vi "cDAQ_VI_Leo_ControlLoop.vi"() -> ()   [LabVIEW 2022 SP3]
uses:
  <vilib>/Analysis/baseanly.llb/Mean (DBL).vi
  STOP_GLOBAL.vi
  <vilib>/DAQmx/miscellaneous.llb/DAQmx Fill In Error Info.vi
  <vilib>/DAQmx/configure/timing.llb/DAQmx Timing (Sample Clock).vi
  <vilib>/DAQmx/read.llb/DAQmx Read (Analog 1D Wfm NChan NSamp).vi
  <vilib>/Analysis/NI_AALBase.lvlib
  <vilib>/addons/control/pid/NI_PID_pid.lvlib
  <vilib>/ptbypt/NI_PtbyPt.lvlib
  <vilib>/addons/control/pid/pid.llb/PID (DBL).vi
panel:
  out "Gauge":cluster{dbl, dbl}(knob) scale=0.0..10.0
  in  "Setpoint":dbl(slide) scale=0.0..10.0
  in  "Output Range":cluster{"output high":dbl, "output low":dbl}={"output high"=100.0, "output low"=-100.0} {"output low" format="%.2f"; "output high" format="%.2f"}
  in  "PID gains":T1={"proportional gain (Kc)"=1.0, "integral time (Ti, min)"=0.01, "derivative time (Td, min)"=0.0} {"derivative time (Td, min)" format="%.3f"; "integral time (Ti, min)" format="%.3f"; "proportional gain (Kc)" format="%.3f"}
  out "element 2":dbl
  out "Array 2":dbl[](array[numeric])
  out "size(s)":i32
  out "Array":dbl[](array[numeric])
  in  "rate":dbl=1000.0 format="%0.2f"
  in  "number of samples":i32=100
  in  "File Format":string
  in  "File Name Out":string
  in  "Data Collection Folder":path
  out "Temperature":dbl[](graph)
  out "Temperature":dynamicdata(graph)
  out "Thrust":dbl[](graph)
  out "Numeric 2":i32
  out "Thrust lb":dynamicdata(graph)
  in  "Types of Testing":enum32{"Test Firing", "Cold Flow Rig"}(tab)
  out "Saving Data":bool
  out "Filename Out":path
  in  "Collect Data?":bool=TRUE caption="Enable"
  in  "Collect Data? 2":bool=TRUE caption="Enable"
  out "Saving Data":bool
  out "Filename Out":path
  out "Supply Pressure PSI":dynamicdata(graph)
  out "4th Channel NI 9219":dynamicdata(graph)
  out "Mass Flow":dbl[](graph)
  out "Mass Flow L/min":dynamicdata(graph)
  out "Chamber Pressure":dbl[](graph)
  out "Supply Pressure":dbl[](graph)
  out "Chamber Pressure PSI":dynamicdata(graph)
  # "DATA LOGGING INFORMATION"
  # "ANALOG VOLTAGE OUTPUT"
  # "RESULTS"
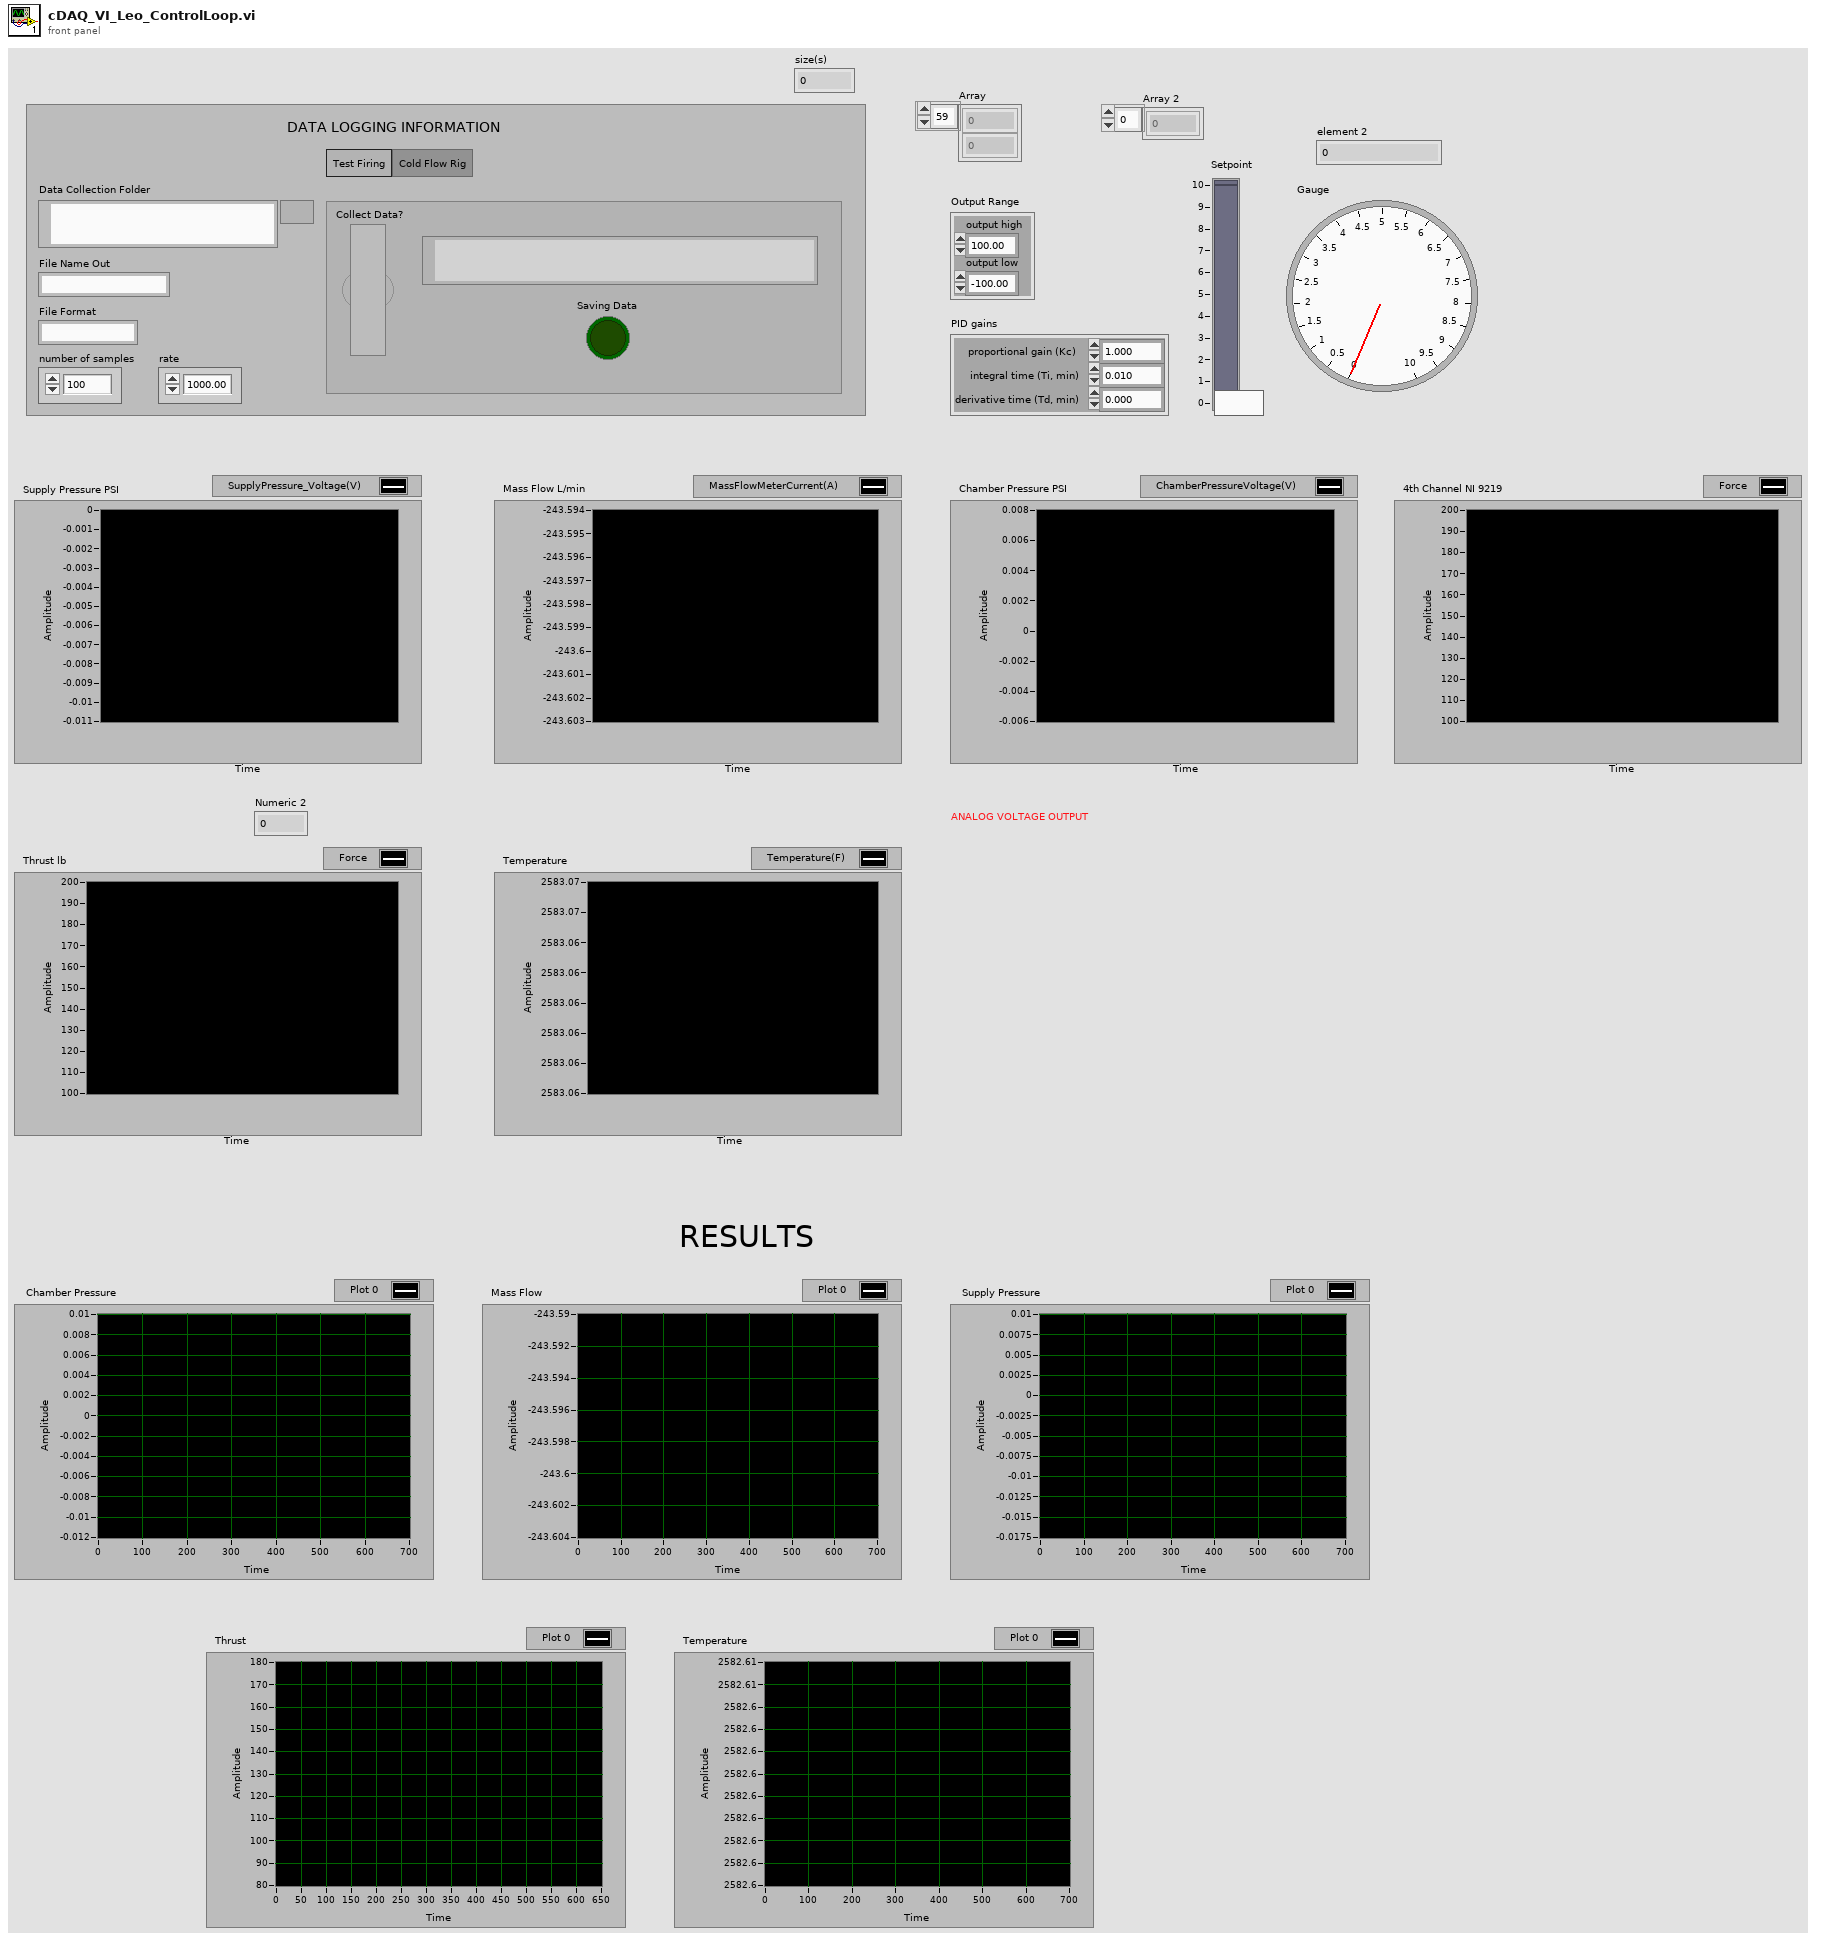
[diagram p1: front panel]
types:
  T1 = cluster{"proportional gain (Kc)":dbl, "integral time (Ti, min)":dbl, "derivative time (Td, min)":dbl}
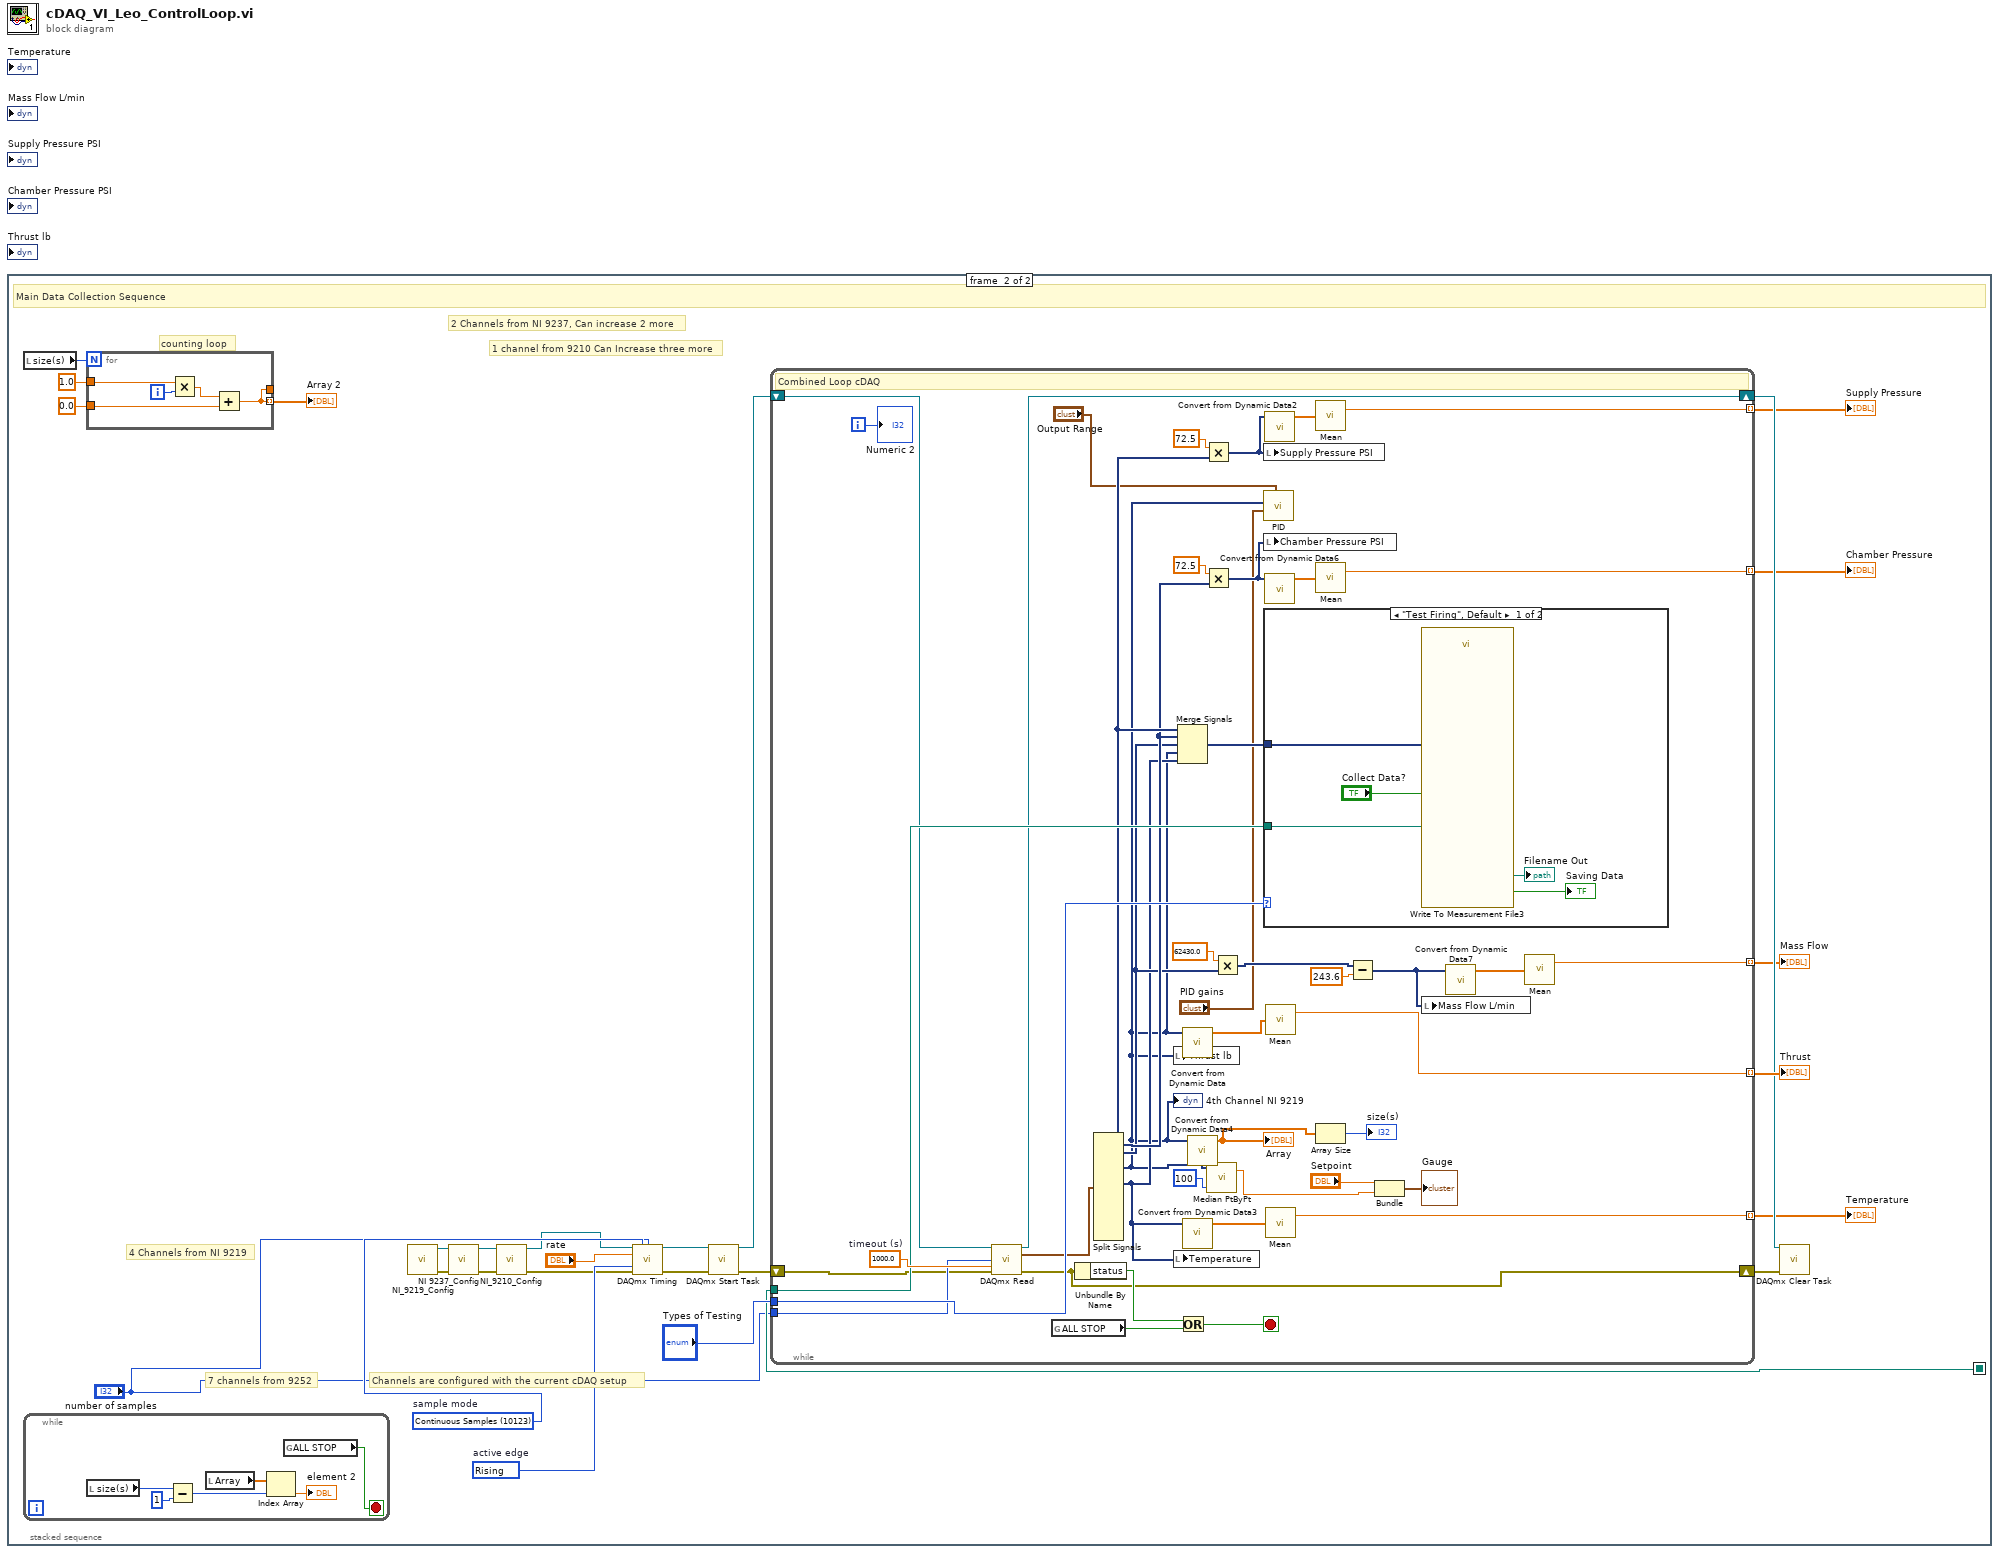
[diagram p0: block diagram]
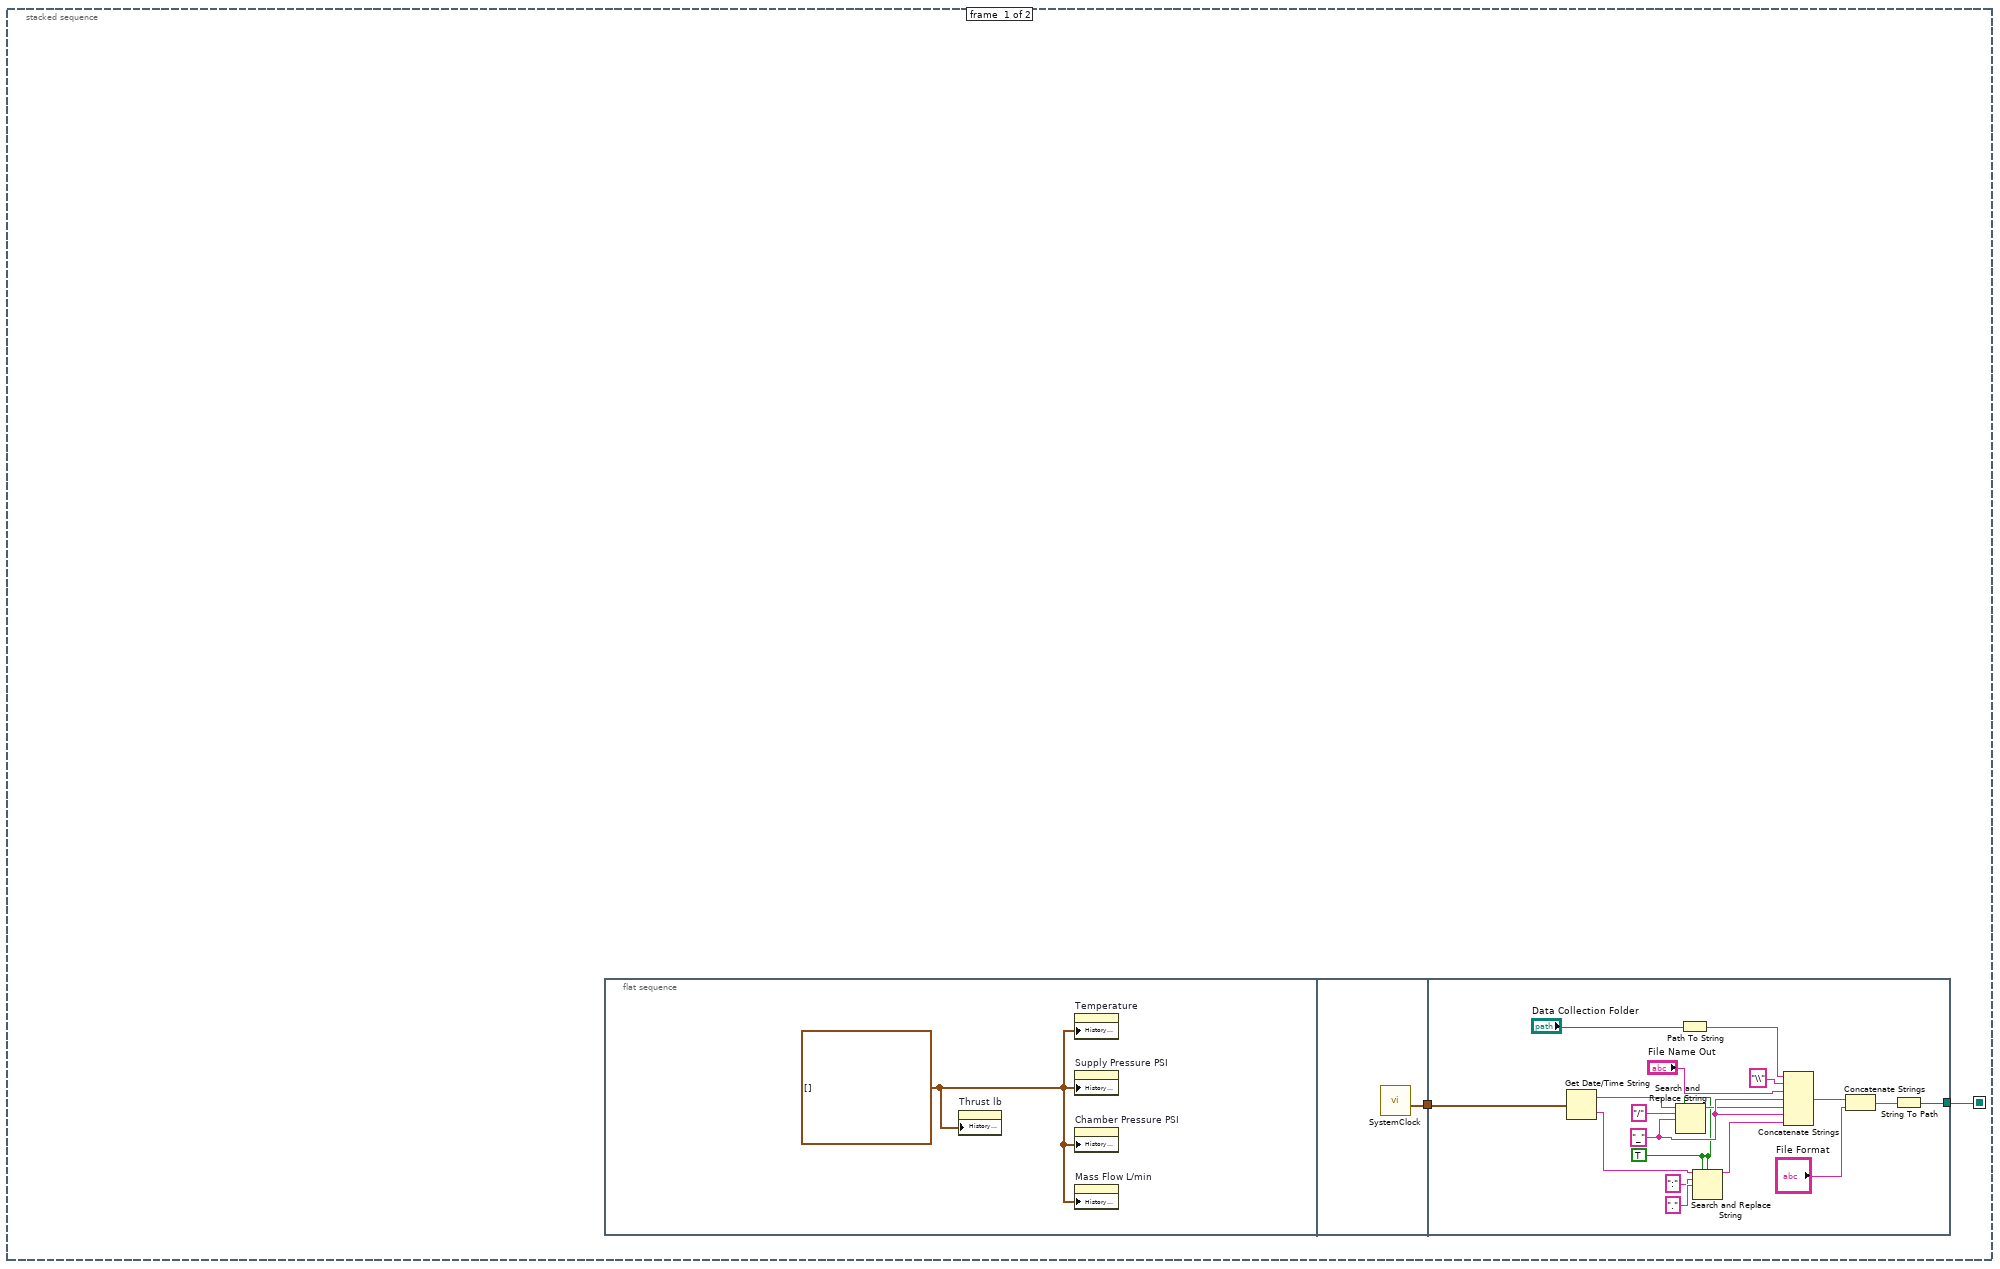
[diagram p2: hidden frame]
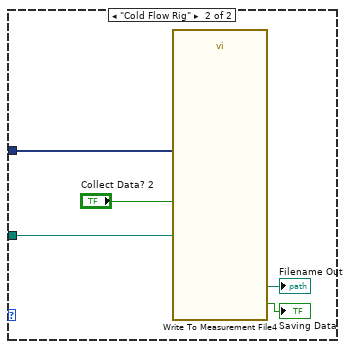
[diagram p3: hidden frame]
diagram:
  n1 = stacked-sequence {
    seq-local: [w1 _] -> [_ w47]
    frame #0 {
      n2 = flat-sequence {
        tunnel: [w4] -> w2
        tunnel: w2 -> [w11]
        tunnel: [w10] -> w1
        frame #0 {
          w3 = waveform(dbl)[] []
          n3 = property on="Thrust lb" class="WFChart (strict)"("History Data"=w3) -> ()  [unwired: 2 in, 2 out]
          n4 = property on="Temperature" class="WFChart (strict)"("History Data"=w3) -> ()  [unwired: 2 in, 2 out]
          n5 = property on="Supply Pressure PSI" class="WFChart (strict)"("History Data"=w3) -> ()  [unwired: 2 in, 2 out]
          n6 = property on="Chamber Pressure PSI" class="WFChart (strict)"("History Data"=w3) -> ()  [unwired: 2 in, 2 out]
          n7 = property on="Mass Flow L/min" class="WFChart (strict)"("History Data"=w3) -> ()  [unwired: 2 in, 2 out]
        }
        frame #1 {
          n8 = call "SystemClock.vi"() -> ("LabVIEW Time Stamp"=w4:timestamp)  [unwired: 9 in, 2 out]
        }
        frame #2 {
          w6 = TRUE ("replace all? (F)")
          w19 = "_" ("string")
          n9 = Get Date/Time String(seconds (now)=w11) -> (date string=w13:string, time string=w16:string)  [unwired: 2 in]
          n10 = Search and Replace String(replace all?=w6, input string=w13, search string="/", replace string=w19) -> (result string=w15:string)  [unwired: 4 in, 3 out]
          n11 = Path To String(path="Data Collection Folder") -> (string=w8:string)
          n12 = Search and Replace String(replace all?=w6, case sensitive?=w6, input string=w16, search string=":", replace string="." ("replace string (\"\")")) -> (result string=w20:string)  [unwired: 3 in, 3 out]
          n13 = Concatenate Strings(w8, "\\" ("string"), "File Name Out", w19, w15, w19, w20) -> (w21:string)
          n14 = Concatenate Strings(w21, "File Format") -> (w22:string)
          n15 = String To Path(string=w22) -> (path=w10:path)
        }
      }
    }
    frame #1 {
      w45 = 10123 items=["Finite Samples"=10178, "Continuous Samples"=10123, "Hardware Timed Single Point"=12522]  # sample mode
      w46 = 10280 items=["Rising"=10280, "Falling"=10171]  # active edge
      # "counting loop"
      # "Channels are configured with the current cDAQ setup"
      # "7 channels from 9252"
      # "1 channel from 9210 Can Increase three more"
      # "2 Channels from NI 9237, Can increase 2 more"
      # "4 Channels from NI 9219"
      # "Main Data Collection Sequence"
      n16 = local read "size(s)"() -> (w25:i32)
      n17 = while {
        stop <- w55 stop-if-true
        n18 = local read "size(s)"() -> (w54:i32)
        n19 = Subtract(x=w54, y=1 ("y 3")) -> (x-y=w53:i32)
        n20 = local read "Array"() -> (w51:dbl[])
        n21 = Index Array(array=w51, index=w53) -> (element=→"element 2":dbl)
        n22 = global read "STOP_GLOBAL.vi" "ALL STOP"() -> (w55:bool)
      }
      n23 = for {
        N: w25 -> [_]
        tunnel: 1.0 ("x") -> [w60]
        tunnel: 0.0 ("y") -> [w57]
        tunnel: [w56] -> w26 mode=indexing
        tunnel: [w56] -> _
        i -> [w59]
        n24 = Multiply(x=w60, y=w59) -> (x*y=w58:dbl)
        n25 = Add(x=w58, y=w57) -> (x+y=w56:dbl)
      }
      "Array 2" <- w26
      n26 = call "NI_9219_Config.vi"() -> ("error out"=w38:errorcluster, "task out"=w37:refnum<k21>)  [unwired: 10 in]
      n27 = call "NI 9237_Config.vi"("error in"=w38, "task in"=w37) -> ("error out"=w35:errorcluster, "task out"=w36:refnum<k21>)  [unwired: 8 in]
      n28 = call "NI_9210_Config.vi"("error in"=w35, "task in"=w36) -> ("error out"=w23:errorcluster, "task out"=w24:refnum<k21>)  [unwired: 8 in]
      n29 = call-poly <vilib>:"DAQmx Timing.vi"("task/channels in"=w24, "sample mode"=w45, "samples per channel"="number of samples", "rate"="rate", "active edge"=w46, "error in"=w23) -> ("task out"=w44:refnum<k21>, "error out"=w43:errorcluster)  [unwired: 8 in]
      n30 = call <vilib>:"DAQmx Start Task.vi"("task/channels in"=w44, "error in"=w43) -> ("task out"=w42:refnum<k21>, "error out"=w41:errorcluster)  [unwired: 12 in]
      n31 = while {
        tunnel: "Types of Testing" -> [w104]
        tunnel: [w102] -> w49 mode=indexing
        tunnel: w47 -> [w97]
        tunnel: "number of samples" -> [w95]
        shift-right: [w91] -> w39
        shift-left: w41 -> [w94]
        shift-right: [w92] -> w40
        shift-left: w42 -> [w93]
        tunnel: [w85] -> w34 mode=indexing
        tunnel: [w82] -> w33 mode=indexing
        tunnel: [w80] -> w32 mode=indexing
        tunnel: [w74] -> w31 mode=indexing
        i -> [w105]
        stop <- w98 stop-if-true
        w100 = 1000.0  # timeout (s)
        # "Combined Loop cDAQ"
        n32 = call-poly <vilib>:"DAQmx Read.vi"("task/channels in"=w93, "number of samples per channel"=w95, "timeout"=w100, "error in"=w94) -> ("task out"=w92:refnum<k21>, "data"=w96:waveform(dbl)[], "error out"=w91:errorcluster)  [unwired: 9 in]
        n33 = global read "STOP_GLOBAL.vi" "ALL STOP"() -> (w99:bool)
        n34 = Unbundle By Name(w91) -> ("status"=w101:bool)
        n35 = Split Signals(w96) -> (w79:dynamicdata, w78:dynamicdata, w77:dynamicdata, w65:dynamicdata, w70:dynamicdata)  [unwired: 14 in, 9 out]
        "4th Channel NI 9219" <- w65
        n36 = local write "Thrust lb"(w65) -> ()
        n37 = local write "Temperature"(w70) -> ()
        n38 = Merge Signals(w79, w78, w77, w65, w70) -> (w76:dynamicdata)
        n39 = Or(x=w101, y=w99) -> (x .or. y?=w98:bool)
        n40 = call "Convert from Dynamic Data"("Dynamic Data Type"=w65) -> ("Array"=w103:dbl[])  [unwired: 3 in]
        n41 = call "Convert from Dynamic Data3"("Dynamic Data Type"=w70) -> ("Array"=w75:dbl[])  [unwired: 3 in]
        n42 = call "Convert from Dynamic Data4"("Dynamic Data Type"=w65) -> ("Array"=w68:dbl[])  [unwired: 3 in]
        "Array" <- w68
        n43 = Multiply(x=72.5, y=w79) -> (x*y=w71:dynamicdata)
        n44 = Multiply(x=72.5, y=w78) -> (x*y=w73:dynamicdata)
        n45 = call <vilib>:"Median PtByPt.vi"("sample length"=100, "x"=w65) -> ("median"=w63:dbl)  [unwired: 2 in, 1 out]
        n46 = Multiply(x=62430.0, y=w77) -> (x*y=w87:dynamicdata)
        n47 = local write "Supply Pressure PSI"(w71) -> ()
        n48 = call-poly <vilib>:"PID.vi"("output range"="Output Range", "PID gains"="PID gains", "process variable"=w65) -> ()  [unwired: 7 in, 2 out]
        n49 = local write "Chamber Pressure PSI"(w73) -> ()
        n50 = case shown="\"Test Firing\", Default" w104 {
          tunnel: w97 -> [w108 w112]
          tunnel: w76 -> [w106 w111]
          frame "Test Firing", Default {
            n51 = call "Write To Measurement File3"("Signals"=w106, "Enable"="Collect Data?", "Filename"=w108) -> ("Filename Out"=→"Filename Out":path, "Saving Data"=→"Saving Data":bool)  [unwired: 14 in, 1 out]
          }
          frame "Cold Flow Rig" {
            n52 = call "Write To Measurement File4"("Signals"=w111, "Enable"="Collect Data? 2", "Filename"=w112) -> ("Filename Out"=→"Filename Out":path, "Saving Data"=→"Saving Data":bool)  [unwired: 14 in, 1 out]
          }
        }
        n53 = call "Convert from Dynamic Data2"("Dynamic Data Type"=w71) -> ("Array"=w84:dbl[])  [unwired: 3 in]
        n54 = call "Convert from Dynamic Data6"("Dynamic Data Type"=w73) -> ("Array"=w83:dbl[])  [unwired: 3 in]
        n55 = call-poly <vilib>:"Mean.vi"("X"=w103) -> ("mean"=w102:dbl)  [unwired: 1 out]
        n56 = call-poly <vilib>:"Mean.vi"("X"=w75) -> ("mean"=w74:dbl)  [unwired: 1 out]
        n57 = call-poly <vilib>:"Mean.vi"("X"=w84) -> ("mean"=w85:dbl)  [unwired: 1 out]
        n58 = call-poly <vilib>:"Mean.vi"("X"=w83) -> ("mean"=w82:dbl)  [unwired: 1 out]
        n59 = Array Size(array=w68) -> (size(s)=→"size(s)":i32)
        n60 = Subtract(x=w87, y=243.6) -> (x-y=w72:dynamicdata)
        n61 = Bundle("Setpoint"="Setpoint", "median"=w63) -> (→"Gauge":cluster{"Setpoint":dbl, "median":dbl})  [unwired: 1 in]
        n62 = local write "Mass Flow L/min"(w72) -> ()
        n63 = call "Convert from Dynamic Data7"("Dynamic Data Type"=w72) -> ("Array"=w81:dbl[])  [unwired: 3 in]
        n64 = call-poly <vilib>:"Mean.vi"("X"=w81) -> ("mean"=w80:dbl)  [unwired: 1 out]
        "Numeric 2" <- w105
      }
      "Supply Pressure" <- w34
      "Chamber Pressure" <- w33
      "Mass Flow" <- w32
      "Thrust" <- w49
      "Temperature" <- w31
      n65 = call <vilib>:"DAQmx Clear Task.vi"("task in"=w40, "error in"=w39) -> ()  [unwired: 13 in, 1 out]
    }
  }
